vi "Test Threshold.vi"(8 "error in (no error)":errorcluster, 11 "Test Case In":refnum<class "Image.lvclass">) -> (0 "error out":errorcluster, 3 "Test Case Out":refnum<class "Image.lvclass">)   [LabVIEW 2020, in "g_ar_toolkit.test.lvlib" / "Image.lvclass"]
uses:
  Image.lvclass
  C:/Program Files (x86)/National Instruments/LabVIEW 2020/vi.lib/Astemes/LUnit/Test Case.lvclass
  g_ar_toolkit.image/Kernel Block Size.ctl
  <vilib>/Astemes/LUnit/Test Case.lvclass/Test Case.ctl
  g_ar_toolkit.image/CreateEmptyImageGreyscale.vi
  g_ar_toolkit.image/CopyArrayToImageGreyscale.vi
  g_ar_toolkit.image/ThresholdBinary.vi
  g_ar_toolkit.image/ThresholdOtsu.vi
  g_ar_toolkit.image/AdaptiveThresholdGaussian.vi
  g_ar_toolkit.image/AdaptiveThresholdMean.vi
  4993e8ee-a06a-463a-9684-69129f64d5ce.vi
  b0764baf-9b14-449e-8268-5b0879581bce.vi
  a2bfb5ea-822a-4dd1-bd6e-1439090374d0.vi
  17070464-f7f7-4e1b-b3d1-8fa198429fcc.vi
  g_ar_toolkit.image/CreateEmptyImageGreyscale.vi/6598b9e0-8a08-46f5-91fd-ca1b87217137.vi
  g_ar_toolkit.image/CopyArrayToImageGreyscale.vi/26c70cee-9332-41f4-9755-08948a885cbe.vi
  g_ar_toolkit.image/ThresholdCore.vi
  g_ar_toolkit.image/AdaptiveThreshold.vi
  <vilib>/Astemes/LUnit/Append Pass Result.vi
  <vilib>/Astemes/LUnit/Append Fail Result.vi
  <vilib>/Astemes/LUnit/Describe Comparison.vi
  <vilib>/Astemes/LUnit/Compare Variants.vi
  <vilib>/Astemes/LUnit/Run In UI.vi
  <vilib>/Utility/error.llb/Clear Errors.vi
  g_ar_toolkit.common/Module Path.vi
  <vilib>/Utility/error.llb/Error Cluster From Error Code.vi
  <vilib>/Astemes/LUnit/Describe Variant.vi
  Image.lvclass/Image.ctl
  g_ar_toolkit.image/g_ar_toolkit.image.lvlib
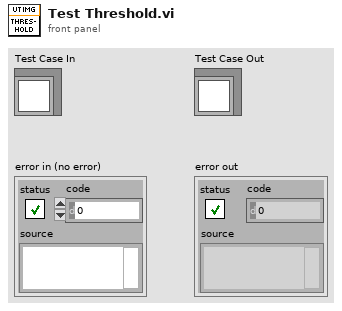
[diagram p1: front panel]
types:
  T1 = typedef "g_ar_toolkit.image.lvlib/Kernel Block Size.ctl" = enum16{"3", "5", "7", "9", "11", "13", "15", "17", "19", "21", "23", "25", "27", "29", "31", "33", "35", "37", "39", "41", "43", "45", "47", "49", "51", "53", "55", "57", "59", "61", "63", "65", "67", "69", "71", "73", "75", "77", "79", "81", "83", "85", "87", "89", "91", "93", "95", "97", "99", "101", "103", "105", "107", "109", "111", "113", "115", "117", "119", "121", "123", "125", "127", "129", "131", "133", "135", "137", "139", "141", "143", "145", "147", "149", "151", "153", "155", "157", "159", "161", "163", "165", "167", "169", "171", "173", "175", "177", "179", "181", "183", "185", "187", "189", "191", "193", "195", "197", "199", "201", "203", "205", "207", "209", "211", "213", "215", "217", "219", "221", "223", "225", "227", "229", "231", "233", "235", "237", "239", "241", "243", "245", "247", "249", "251", "253", "255", "257", "259", "261", "263", "265", "267", "269", "271", "273", "275", "277", "279", "281", "283", "285", "287", "289", "291", "293", "295", "297", "299", "301", "303", "305", "307", "309", "311", "313", "315", "317", "319", "321", "323", "325", "327", "329", "331", "333", "335", "337", "339", "341", "343", "345", "347", "349", "351", "353", "355", "357"}
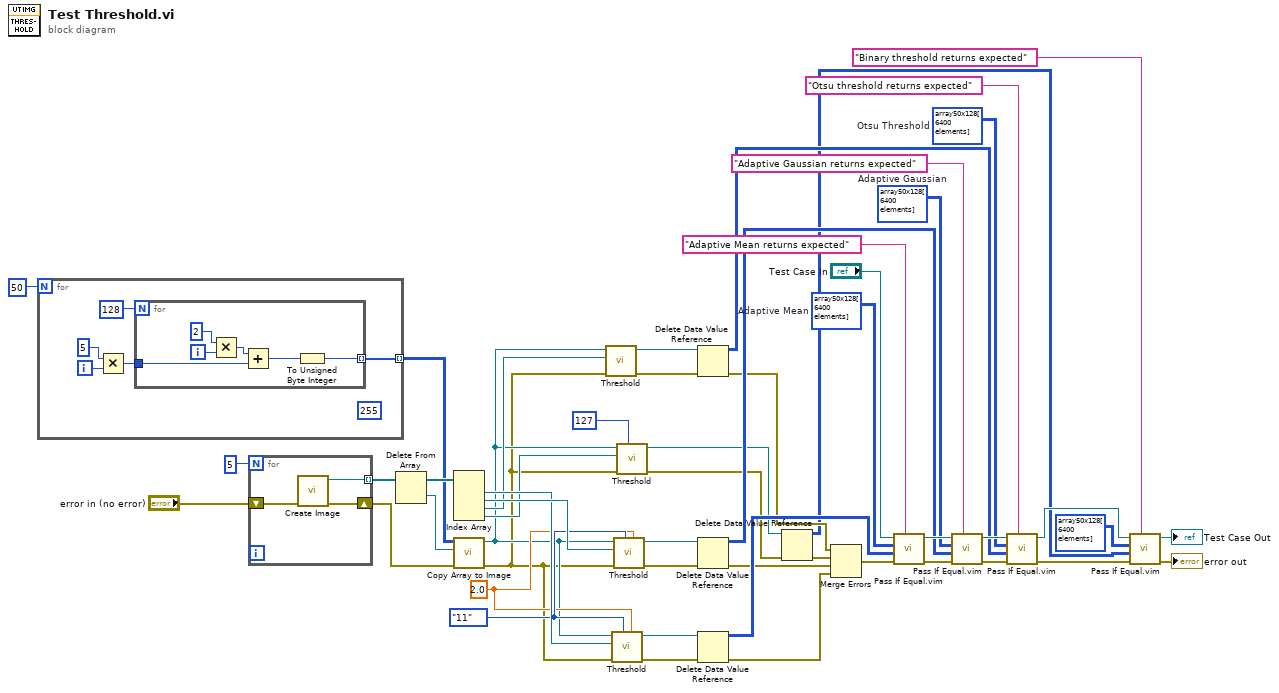
[diagram p0: block diagram]
diagram:
  w28 = u8[][] array50x128[6400 elements]  # Otsu Threshold
  w29 = u8[][] array50x128[6400 elements]  # Adaptive Gaussian
  w32 = u8[][] array50x128[6400 elements]  # Adaptive Mean
  w33 = Kernel_Block_Size."11" ("Kernel Block Size (Default: 5)")
  w18 = 2.0 ("C")
  n1 = for {
    N: 50 -> [_]
    tunnel: [w52] -> w34 mode=indexing
    i -> [w55]
    (unwired) 255
    n2 = Multiply(x=5, y=w55) -> (x*y=w53:i32)
    n3 = for {
      N: 128 -> [_]
      tunnel: w53 -> [w59]
      tunnel: [w57] -> w52 mode=indexing
      i -> [w61]
      n4 = Multiply(x=2, y=w61) -> (x*y=w60:i32)
      n5 = Add(x=w60, y=w59) -> (x+y=w58:i32)
      n6 = To Unsigned Byte Integer(number=w58) -> (unsigned 8bit integer=w57:u8)
    }
  }
  n7 = for {
    N: 5 -> [_]
    tunnel: [w65] -> w49 mode=indexing
    shift-right: [w64] -> w48
    shift-left: "error in (no error)" -> [w63]
    n8 = call-poly "Create Image.vi"("error in (no error)"=w63) -> ("error out"=w64:errorcluster, "New Greyscale Image"=w65:refnum<data-value>)  [unwired: 9 in]
  }
  n9 = Delete From Array(array=w49) -> (deleted portion=w45:refnum<data-value>, array with subset deleted=w44:refnum<data-value>[])  [unwired: 2 in]
  n10 = Index Array(array=w44) -> (element #1=w42:refnum<data-value>, element #2=w43:refnum<data-value>, element #3=w41:refnum<data-value>, element #4=w17:refnum<data-value>)  [unwired: 4 in]
  n11 = call-poly "Copy Array to Image.vi"("error in (no error)"=w48, "Greyscale Destination Image"=w45, "Source"=w34) -> ("error out"=w15:errorcluster, "Greyscale Destination Image (duplicate)"=w16:refnum<data-value>)  [unwired: 7 in]
  n12 = call-poly "Threshold.vi"("error in (no error)"=w15, "Otsu Threshold Result"=w41, "Greyscale Image-Source"=w16) -> ("error out"=w36:errorcluster, "Otsu Threshold Result (duplicate)"=w35:refnum<data-value>)  [unwired: 7 in]
  n13 = call-poly "Threshold.vi"("C"=w18, "Kernel Block Size (Default: 5)"=w33, "error in (no error)"=w15, "Adaptive Threshold Result"=w42, "Greyscale Image-Source"=w16) -> ("error out"=w40:errorcluster, "Adaptive Threshold Result (duplicate)"=w39:refnum<data-value>)  [unwired: 5 in]
  n14 = call-poly "Threshold.vi"("C"=w18, "Kernel Block Size (Default: 5)"=w33, "error in (no error)"=w15, "Adaptive Threshold Result"=w43, "Greyscale Image-Source"=w16) -> ("error out"=w38:errorcluster, "Adaptive Threshold Result (duplicate)"=w37:refnum<data-value>)  [unwired: 5 in]
  n15 = call-poly "Threshold.vi"("Threshold"=u8 127, "error in (no error)"=w15, "Threshold Result"=w17, "Greyscale Image-Source"=w16) -> ("error out"=w13:errorcluster, "Threshold Result (duplicate)"=w12:refnum<data-value>)  [unwired: 6 in]
  n16 = Delete Data Value Reference(data value reference=w35, error in=w36) -> (data value=w27:u8[][], error out=w14:errorcluster)
  n17 = Delete Data Value Reference(data value reference=w37, error in=w38) -> (data value=w26:u8[][], error out=w10:errorcluster)
  n18 = Delete Data Value Reference(data value reference=w39, error in=w40) -> (data value=w25:u8[][], error out=w9:errorcluster)
  n19 = Delete Data Value Reference(data value reference=w12, error in=w13) -> (data value=w3:u8[][], error out=w11:errorcluster)
  n20 = Merge Errors(w14, w11, w10, w9) -> (w8:errorcluster)
  n21 = call "Pass If Equal.vim"("Description"="Adaptive Mean returns expected", "error in (no error)"=w8, "Actual"=w25, "Expected"=w32, "LUnit Test Case In"="Test Case In") -> ("error out"=w24:errorcluster, "LUnit Test Case Out"=w31:refnum<class "Image.lvclass">)  [unwired: 5 in]
  n22 = call "Pass If Equal.vim"("Description"="Adaptive Gaussian returns expected", "error in (no error)"=w24, "Actual"=w26, "Expected"=w29, "LUnit Test Case In"=w31) -> ("error out"=w23:errorcluster, "LUnit Test Case Out"=w30:refnum<class "Image.lvclass">)  [unwired: 5 in]
  n23 = call "Pass If Equal.vim"("Description"="Otsu threshold returns expected", "error in (no error)"=w23, "Actual"=w27, "Expected"=w28, "LUnit Test Case In"=w30) -> ("error out"=w22:errorcluster, "LUnit Test Case Out"=w5:refnum<class "Image.lvclass">)  [unwired: 5 in]
  n24 = call "Pass If Equal.vim"("Description"="Binary threshold returns expected", "error in (no error)"=w22, "Actual"=w3, "Expected"=u8[][] array50x128[6400 elements] ("data value"), "LUnit Test Case In"=w5) -> ("error out"=→"error out":errorcluster, "LUnit Test Case Out"=→"Test Case Out":refnum<class "Image.lvclass">)  [unwired: 5 in]
